vi "REV2mDistanceSensor Close.vi"(8 "error in (no error)":errorcluster, 11 "REV2mDistanceSensorsArray":T1={"Automatic Enabled"=TRUE, "Sensors[]"=[]}) -> (0 "error out":errorcluster)   [LabVIEW 2019, in "DistanceSensorDriver.lvlib"]
uses:
  DistanceSensorDriver.lvlib
  Typedef/Rev2mDistanceSensorsArray.ctl
  Typedef/REV2mDistanceSensorDevRef.ctl
  Typedef/Ports.ctl
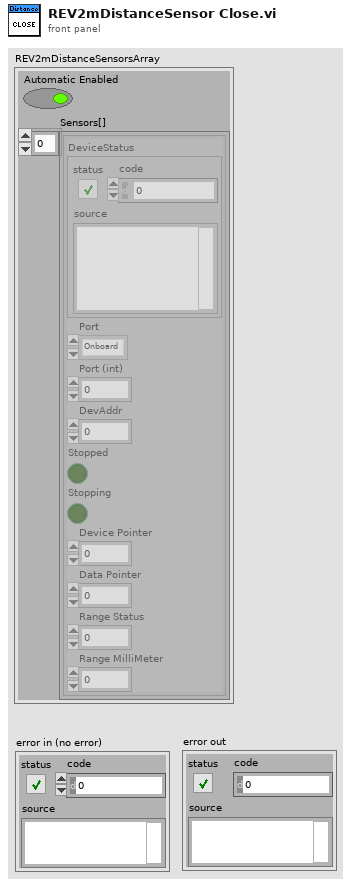
[diagram p1: front panel]
types:
  T1 = typedef "DistanceSensorDriver.lvlib/Rev2mDistanceSensorsArray.ctl" = cluster{"Automatic Enabled":bool, "Sensors[]":T2[]}
  T2 = typedef "DistanceSensorDriver.lvlib/REV2mDistanceSensorDevRef.ctl" = cluster{"DeviceStatus":errorcluster, "Port":T3, "Port (int)":i32, "DevAddr":i32, "Stopped":bool, "Stopping":bool, "Device Pointer":u64, "Data Pointer":u64, "Range Status":u8, "Range MilliMeter":u16}
  T3 = typedef "DistanceSensorDriver.lvlib/Ports.ctl" = enum32{"Onboard", "MXP"}
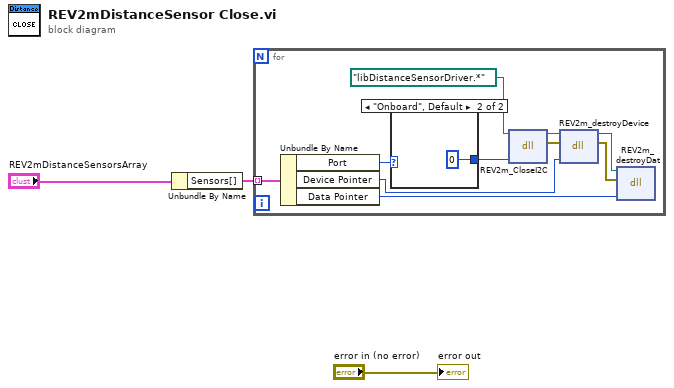
[diagram p0: block diagram]
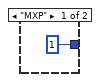
[diagram p2: hidden frame]
diagram:
  n1 = Unbundle By Name("REV2mDistanceSensorsArray") -> ("Sensors[]"=w1:T2[])
  n2 = for {
    tunnel: w1 -> [w10] mode=indexing
    n3 = Unbundle By Name(w10) -> ("Port"=w12:T3, "Device Pointer"=w7:u64, "Data Pointer"=w4:u64)
    n4 = case shown="\"Onboard\", Default" w12 {
      tunnel: [1 ("port") 0 ("port")] -> w11
      frame "MXP" {
      }
      frame "Onboard", Default {
      }
    }
    n5 = dll-call lib="?" fn="REV2m_CloseI2C"(path in=path "libDistanceSensorDriver.*", "port"=w11) -> (path out=w9:path, error out=w8:errorcluster)  [unwired: 4 in]
    n6 = dll-call lib="?" fn="REV2m_destroyDevice"(path in=w9, error in=w8, "Dev"=w7) -> (path out=w6:path, error out=w5:errorcluster)  [unwired: 3 in]
    n7 = dll-call lib="?" fn="REV2m_destroyDat"(path in=w6, error in=w5, "Dev"=w4) -> ()  [unwired: 3 in, 2 out]
  }
  "error out" <- "error in (no error)"
